vi "ProcessTemplate.vi"(10 "InitString":string, 11 "EVE reference in":refnum<data-value>) -> ()   [LabVIEW 2013, in "Template.lvclass"]
uses:
  Class/Template.lvclass
  001 - MAIN/Class/EVE/EVE.lvclass
  090 - ERRORS/Ctrls/enumLogAndView.ctl
  030 - EVENTS/03 - ToMessageHandlerProcess/ToMessageHandlerEvent.ctl
  030 - EVENTS/03 - ToMessageHandlerProcess/enumMessageCriticity.ctl
  Class/Process/Process.lvclass
panel:
  # "Template de process ..."
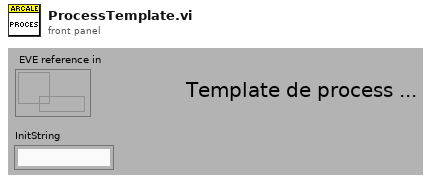
[diagram p1: front panel]
types:
  T1 = typedef "enumLogAndView.ctl" = enum16{"Log only", "Log and view"}
  T2 = typedef "enumMessageCriticity.ctl" = enum16{"No error", "Info", "Warning", "Error", "Fatal error"}
  T3 = typedef "ToMessageHandlerEvent.ctl" = cluster{"date / time":timestamp, "Criticity":T2, "Emitter":string, "Message":string}
  T4 = enum32{"Invalid", "Standard", "Closed", "Hidden", "Minimized", "Maximized"}
  T5 = typedef "EnumToAllProcessesCommand.ctl" = enum16{"Stop all processes", "Autotest"}
  T6 = typedef "ToProcess_EnumCommand.ctl" = enum16{"Show front panel", "Hide front panel"}
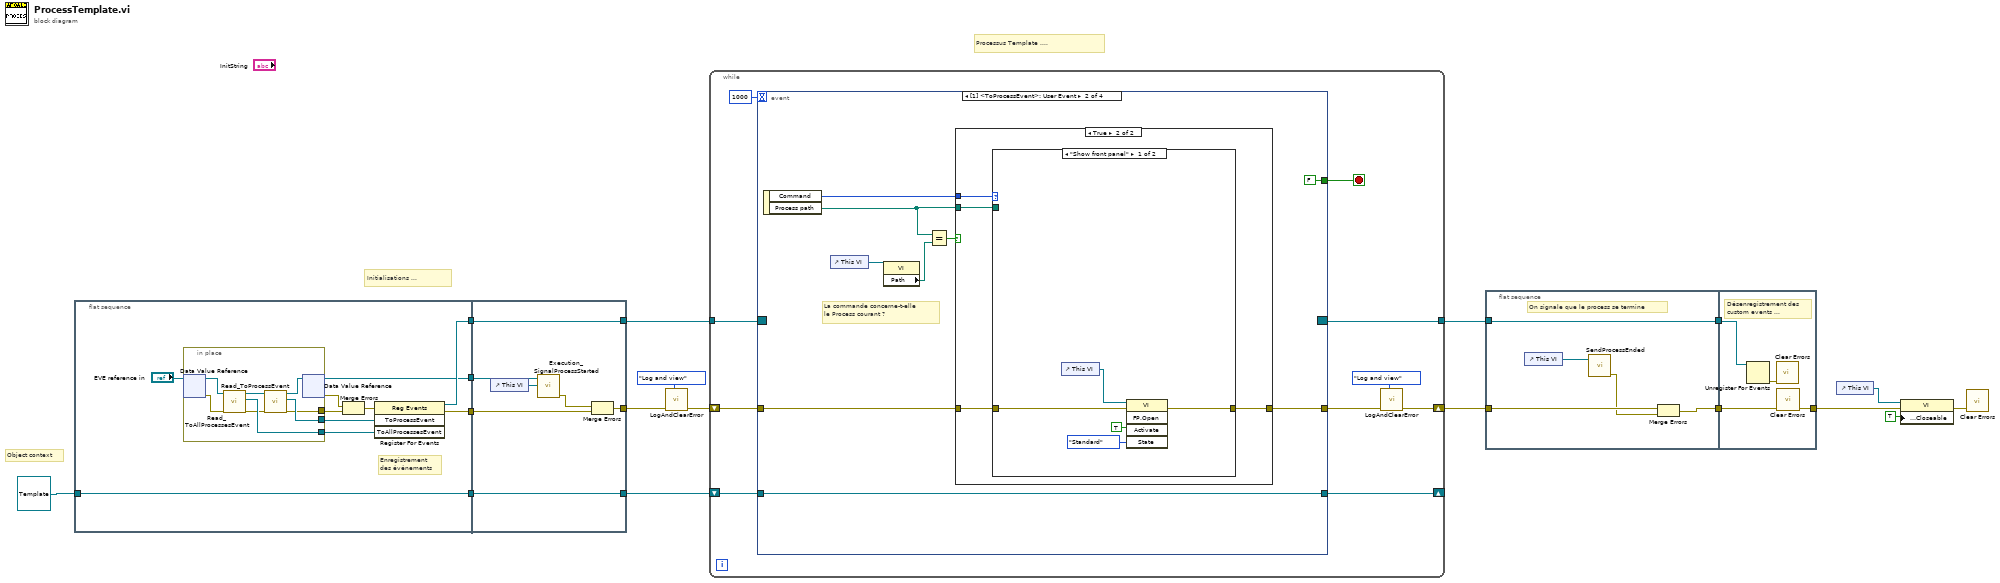
[diagram p0: block diagram]
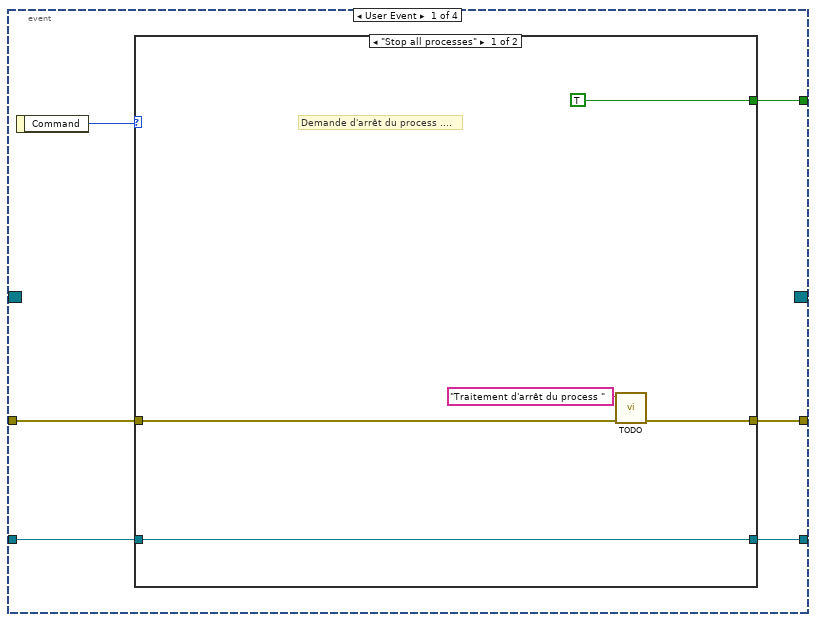
[diagram p2: hidden frame]
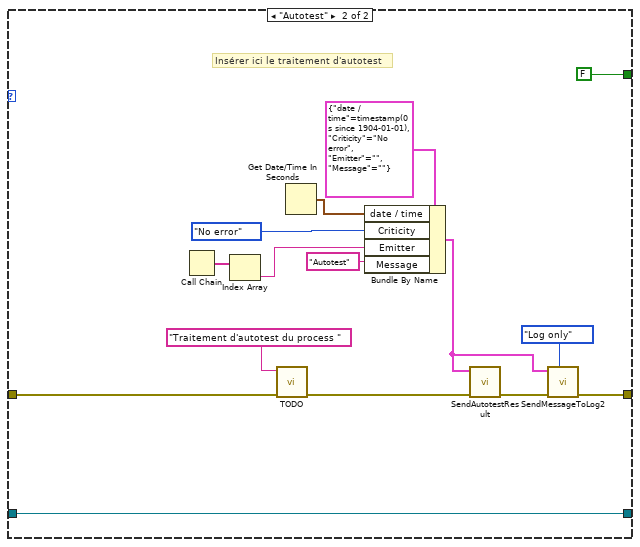
[diagram p3: hidden frame]
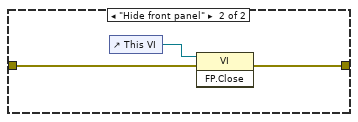
[diagram p5: hidden frame]
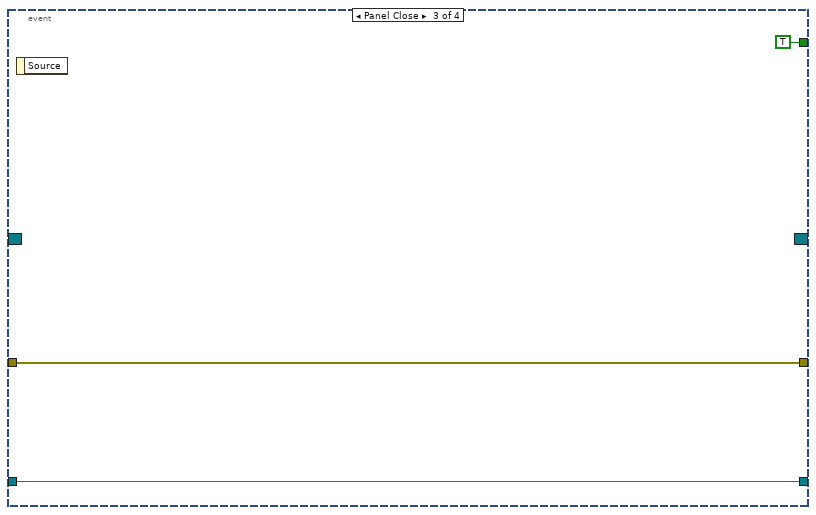
[diagram p6: hidden frame]
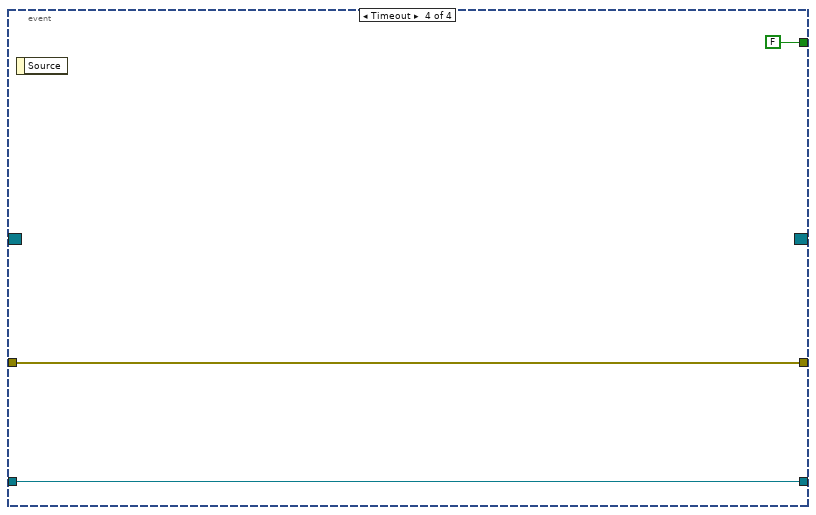
[diagram p7: hidden frame]
diagram:
  # "Object context"
  # "Initialisations ..."
  # "Processus Template ...."
  n1 = flat-sequence {
    tunnel: refnum<class "Template.lvclass"> refnum ("Template.lvclass") -> [w28]
    tunnel: [w28] -> w15
    tunnel: [w27] -> w10
    tunnel: [w26] -> w9
    tunnel: [w19] -> w1
    tunnel: [w43] -> w11
    tunnel: [w41] -> w18
    tunnel: w15 -> [w42]
    tunnel: [w42] -> w14
    tunnel: w10 -> [w40]
    tunnel: w9 -> [w41]
    tunnel: w1 -> [w38]
    frame #0 {
      # "Enregistrement \ndes événements"
      n2 = in-place {
        in-place-border: [w33] -> w24
        in-place-border: [w32] -> w23
        in-place-border: [w29] -> w22
        n3 = in-place-dvr #1("EVE reference in") -> (w36:refnum<class "EVE.lvclass">, w30:errorcluster)
        n4 = call-dynamic "Read_ToAllProcessesEvent.vi"("error in (no error)"=w30, "EVE in"=w36) -> ("error out"=w31:errorcluster, "ToAllProcessesEvent"=w33:refnum<user-event>, "EVE out"=w35:refnum<class "EVE.lvclass">)  [unwired: 7 in]
        n5 = call-dynamic "Read_ToProcessEvent.vi"("error in (no error)"=w31, "EVE in"=w35) -> ("error out"=w29:errorcluster, "ToProcessEvent"=w32:refnum<user-event>, "EVE out"=w34:refnum<class "EVE.lvclass">)  [unwired: 7 in]
        n6 = in-place-dvr #1(w34) -> (w19:refnum<data-value>, w21:errorcluster)
      }
      n7 = Merge Errors(w21, w22) -> (w20:errorcluster)
      n8 = register-events(error in=w20, w23, w24) -> (reference out=w26:refnum<event-registration>, error out=w27:errorcluster)  [unwired: 1 in]
    }
    frame #1 {
      n9 = control-ref of="This VI"() -> (w37:refnum<vi>)
      n10 = call "Execution_SignalProcessStarted.vi"("This VI"=w37, "EVE reference in"=w38) -> ("error out"=w39:errorcluster)  [unwired: 9 in]
      n11 = Merge Errors(w39, w40) -> (w43:errorcluster)
    }
  }
  n12 = call "LogAndClearError.vi"("Log and view ?"=enumLogAndView."Log and view", "error in (no error)"=w11) -> ("error out"=w12:errorcluster)  [unwired: 9 in]
  n13 = while {
    shift-right: [w47] -> w16
    shift-left: w12 -> [w44]
    tunnel: w18 -> [w53]
    tunnel: [w52] -> w17
    shift-right: [w49] -> _
    shift-left: w14 -> [w50]
    stop <- w51 stop-if-true
    n14 = event shown="[1] <ToProcessEvent>: User Event" {
      selector: w53 -> [_ _ _ _]
      dyn-events: [_ _ _ _] -> w52
      timeout: 1000 -> [_ _ _ _]
      tunnel: w44 -> [w57 w87 w103 w107]
      tunnel: [w56 w83 w103 w107] -> w48
      tunnel: [w58 FALSE TRUE FALSE] -> w51
      tunnel: w50 -> [w55 w82 w102 w106]
      tunnel: [w54 w82 w102 w106] -> w49
      event User Event {
        n15 = event-data() -> ("Command"=w59:T5)  [unwired: 1 in]
        n16 = case shown="\"Stop all processes\"" w59 {
          tunnel: [TRUE FALSE] -> w58
          tunnel: w57 -> [w60 w76]
          tunnel: [w62 w67] -> w56
          tunnel: w55 -> [w63 w79]
          tunnel: [w63 w79] -> w54
          frame "Stop all processes" {
            # "Demande d'arrêt du process ...."
            n17 = call "TODO.vi"("error in (no error)"=w60, "Message"="Traitement d'arrêt du process ") -> ("error out"=w62:errorcluster)  [unwired: 9 in]
          }
          frame "Autotest" {
            # "Insérer ici le traitement d'autotest"
            n18 = Call Chain() -> (call chain=w71:string[])
            n19 = Index Array(array=w71) -> (element=w70:string)  [unwired: 1 in]
            n20 = call "TODO.vi"("error in (no error)"=w76, "Message"="Traitement d'autotest du process ") -> ("error out"=w75:errorcluster)  [unwired: 9 in]
            n21 = Get Date/Time In Seconds() -> (seconds since 1Jan1904=w73:timestamp)
            n22 = Bundle By Name(cluster=T3 {"date / time"=timestamp(0 s since 1904-01-01), "Criticity"=enum."No error", "Emitter"="", "Message"=""} ("Message"), "date / time"=w73, "Criticity"=enumMessageCriticity."No error", "Emitter"=w70, "Message"="Autotest") -> (w66:T3)
            n23 = call "SendAutotestResult.vi"("error in (no error)"=w75, "Message"=w66) -> ("error out"=w68:errorcluster)  [unwired: 9 in]
            n24 = call "SendMessageToLog2.vi"("Log and view ?"=enumLogAndView."Log only", "error in (no error)"=w68, "Message"=w66) -> ("error out"=w67:errorcluster)  [unwired: 8 in]
          }
        }
      }
      event User Event {
        # "La commande concerne-t-elle\nle Process courant ?"
        n25 = event-data() -> ("Command"=w88:T6, "Process path"=w85:path)  [unwired: 1 in]
        n26 = control-ref of="This VI"() -> (w86:refnum<vi>)
        n27 = property class="VI"(reference=w86) -> ("Path"=w84:path)  [unwired: 1 in, 2 out]
        n28 = Equal?(x=w85, y=w84) -> (x = y?=w81:bool)
        n29 = case shown="True" w81 {
          tunnel: w88 -> [_ w93]
          tunnel: w87 -> [w89 w92]
          tunnel: w85 -> [_ w91]
          tunnel: [w89 w90] -> w83
          frame False {
            # "La commande n'est pas pour ce process !"
          }
          frame True {
            n30 = case shown="\"Show front panel\"" w93 {
              tunnel: w92 -> [w97 w100]
              tunnel: w91 -> [_ _]
              tunnel: [w96 w99] -> w90
              frame "Show front panel" {
                n31 = control-ref of="This VI"() -> (w98:refnum<vi>)
                n32 = invoke class="VI" method="FP.Open"(reference=w98, error in=w97, "Activate"=TRUE ("Activate?"), "State"=T4."Standard") -> (error out=w96:errorcluster)  [unwired: 1 in, 4 out]
              }
              frame "Hide front panel" {
                n33 = control-ref of="This VI"() -> (w101:refnum<vi>)
                n34 = invoke class="VI" method="FP.Close"(reference=w101, error in=w100) -> (error out=w99:errorcluster)  [unwired: 1 in, 2 out]
              }
            }
          }
        }
      }
      event Panel Close {
        n35 = event-data() -> ()  [unwired: 1 in, 1 out]
      }
      event Timeout {
        n36 = event-data() -> ()  [unwired: 1 in, 1 out]
      }
    }
    n37 = call "LogAndClearError.vi"("Log and view ?"=enumLogAndView."Log and view", "error in (no error)"=w48) -> ("error out"=w47:errorcluster)  [unwired: 9 in]
  }
  n38 = flat-sequence {
    tunnel: w16 -> [w111]
    tunnel: w17 -> [w112]
    tunnel: [w112] -> w4
    tunnel: [w109] -> w3
    tunnel: [w113] -> w8
    tunnel: w4 -> [w116]
    tunnel: w3 -> [w114]
    frame #0 {
      # "On signale que le process se termine"
      n39 = control-ref of="This VI"() -> (w108:refnum<vi>)
      n40 = call "SendProcessEnded.vi"("Process Refnum"=w108) -> ("error out"=w110:errorcluster)  [unwired: 10 in]
      n41 = Merge Errors(w111, w110) -> (w109:errorcluster)
    }
    frame #1 {
      # "Désenregistrement des\ncustom events ..."
      n42 = Unregister For Events(event registration refnum=w116) -> (error out=w115:errorcluster)  [unwired: 1 in]
      n43 = call <vilib>:"Clear Errors.vi"("error in (no error)"=w115) -> ()  [unwired: 6 in, 1 out]
      n44 = call <vilib>:"Clear Errors.vi"("error in (no error)"=w114) -> ("error out"=w113:errorcluster)  [unwired: 6 in]
    }
  }
  n45 = control-ref of="This VI"() -> (w7:refnum<vi>)
  n46 = property class="VI"(reference=w7, error in=w8, "Front Panel.Closeable"=TRUE ("Front Panel Window:Closeable")) -> (error out=w5:errorcluster)  [unwired: 1 out]
  n47 = call <vilib>:"Clear Errors.vi"("error in (no error)"=w5) -> ()  [unwired: 6 in, 1 out]
